vi "MotorBlock_P.vi"(0 "P":dbl, 3 "STOP":bool, 5 "Value":dbl, 7 "Friction Compensation":dbl=0.09 format="%#_13g", 9 "Speed\n (Lower than 900 counts/s)":dbl, 11 "error in (no error)":errorcluster, 12 "Enum":T2(ring), 13 "Motor":T1(ring), 14 "(Antihorario) Sentido (Horario)":bool) -> (4 "Waveform \nChart":dbl[][](graph), 15 "error out":errorcluster)   [LabVIEW 2017]
uses:
  <vilib>/myRIO/Common/Instrument Driver Framework/myRIO v1.0/Encoder/typedefs/Encoder Signal Mode.ctl
  <vilib>/Platform/TimedLoop/XDataNode/timing_clust.ctl
  <vilib>/Platform/TimedLoop/XDataNode/nitl_modes.ctl
  <vilib>/Platform/TimedLoop/XDataNode/wakeup.ctl
  <vilib>/myRIO/Common/Instrument Driver Framework/myRIO v1.0/UART/vis/myRIO v1.0 Close UART.vi
  <vilib>/Utility/error.llb/Error Cluster From Error Code.vi
  <vilib>/myRIO/Common/Instrument Driver Framework/myRIO v1.0/Encoder/vis/myRIO v1.0 Read Encoder.vi
  <vilib>/myRIO/Common/Instrument Driver Framework/myRIO v1.0/DIO/vis/myRIO v1.0 Write DIO.vi
  <vilib>/myRIO/Common/Instrument Driver Framework/myRIO v1.0/PWM/vis/myRIO v1.0 Write PWM.vi
  <vilib>/myRIO/Common/Instrument Driver Framework/Utilities/vis/FPGA Ref Manager.vi
  <vilib>/myRIO/Common/Instrument Driver Framework/myRIO v1.0/myRIO v1.0 Reset FPGA.vi
  <vilib>/myRIO/Common/Instrument Driver Framework/myRIO v1.0/IRQ/vis/myRIO v1.0 IRQ Info FGV.vi
  <vilib>/myRIO/Common/Instrument Driver Framework/myRIO v1.0/IRQ/vis/myRIO v1.0 Timer IRQ Info FGV.vi
  <vilib>/myRIO/Common/Instrument Driver Framework/myRIO v1.0/IRQ/vis/myRIO v1.0 ISR Agent.vi
  <vilib>/Platform/TimedLoop/XDataNode/XDataNode.xnode
  <vilib>/myRIO/Instrument Drivers/Onboard IO/Encoder/Encoder.lvlib
  <vilib>/myRIO/Instrument Drivers/Onboard IO/DIO/DIO.lvlib
  <vilib>/myRIO/Instrument Drivers/Onboard IO/PWM/PWM.lvlib
  <vilib>/myRIO/Instrument Drivers/Utilities/Utilities.lvlib
  <vilib>/Platform/TimedLoop/XDataNode/XDNodeRunTimeDep.lvlib
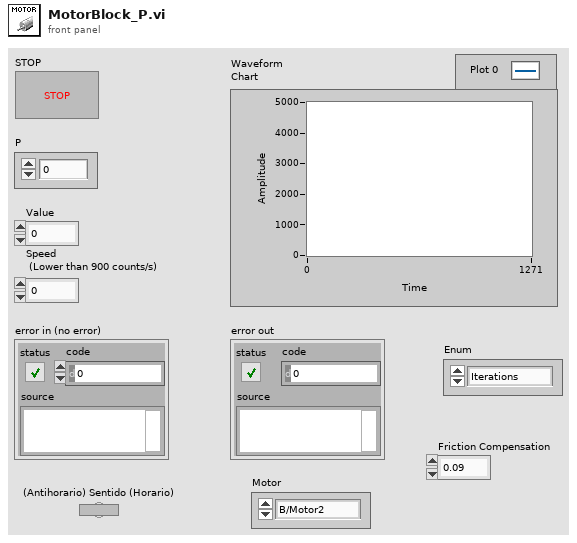
[diagram p1: front panel]
types:
  T1 = enum16{"B/Motor2", "B/Motor1", "A/Motor2", "A/Motor1"}
  T2 = enum16{"Iterations", "Rotations", "Counts", "Degrees", "Time"}
  T3 = typedef "Encoder Signal Mode.ctl" = enum16{"Quadrature phase signal", "Step and direction signal"}
  T4 = typedef "XDNodeRunTimeDep.lvlib/timing_clust.ctl" = cluster{"Expected End [f-1]":u64, "Actual End [f-1]":u64, "Finished Late? [f-1]":bool, "Expected End [i-1]":u64, "Actual End [i-1]":u64, "Finished Late? [i-1]":bool, "Expected Start [i]":u64, "Actual Start [i]":u64, "Expected Start [f]":u64, "Actual Start [f]":u64, "Source Name":string, "Structure Name":string, "Period":i64, "Deadline":i64, "Offset":i64, "Start":i64, "Priority":i32, "Timeout":i32, "Mode":T5, "Wakeup Reason":T6, "Error":errorcluster, "Source Type":string, "Secondary Source Type":string, "Global End Time":u64, "Global Start Time":u64, "Frame Duration":u64, "Iteration Duration":u64, "Assigned CPU":i32, "I/O Scan Engine Mode":u32}
  T5 = typedef "XDNodeRunTimeDep.lvlib/nitl_modes.ctl" = enum32{"No Change", "Process missed periods, maintain original phase", "Discard missed periods, maintain original phase", "Process missed periods, ignore original phase", "Discard missed periods, ignore original phase"}
  T6 = typedef "XDNodeRunTimeDep.lvlib/wakeup.ctl" = enum32{"Normal", "Aborted", "Asynchronous wakeup", "Timing source error", "Timed loop error", "Timeout"}
  T7 = typedef "Encoder.lvlib/Encoder Reference.ctl" = cluster{"myRIO Reference":T8, "Encoder Channels Enum":T12}
  T8 = typedef "myRIO Generic Hardware Reference.ctl" = cluster{"myRIO Model":T9, "myRIO Hardware Reference":T10}
  T9 = typedef "Hardware Version Enum.ctl" = enum16{"Unknown", "myRIO-1900", "myRIO-1950", "roboRIO", "NI ELVIS RIO CM"}
  T10 = typedef "myRIO v1.0 Reference.ctl" = cluster{"Generic FPGA Reference":T11, "Allow multiple opens":bool}
  T11 = typedef "Generic FPGA Reference.ctl" = refnum<k20>
  T12 = typedef "Encoder Channels Enum.ctl" = enum16{"Not Connected", "C/ENC0", "C/ENC1", "A/ENC", "B/ENC", "DIO/ENC0", "DIO/ENC1", "DIO/ENC2", "DIO/ENC3", "DIO/ENC4"}
  T13 = typedef "DIO.lvlib/DIO Reference.ctl" = cluster{"myRIO Reference":T8, "DIO Channels List":T14}
  T14 = typedef "DIO Channels List.ctl" = T15[]
  T15 = typedef "DIO Channels Enum.ctl" = enum16{"Not Connected", "C/DIO0", "C/DIO1", "C/DIO2", "C/DIO3", "C/DIO4", "C/DIO5", "C/DIO6", "C/DIO7", "A/DIO0", "A/DIO1", "A/DIO2", "A/DIO3", "A/DIO4", "A/DIO5", "A/DIO6", "A/DIO7", "A/DIO8", "A/DIO9", "A/DIO10", "A/DIO11", "A/DIO12", "A/DIO13", "A/DIO14", "A/DIO15", "B/DIO0", "B/DIO1", "B/DIO2", "B/DIO3", "B/DIO4", "B/DIO5", "B/DIO6", "B/DIO7", "B/DIO8", "B/DIO9", "B/DIO10", "B/DIO11", "B/DIO12", "B/DIO13", "B/DIO14", "B/DIO15", "LED0", "LED1", "LED2", "LED3", "Button0", "DIO/DIO0", "DIO/DIO1", "DIO/DIO2", "DIO/DIO3", "DIO/DIO4", "DIO/DIO5", "DIO/DIO6", "DIO/DIO7", "DIO/DIO8", "DIO/DIO9", "SPI/CS0", "SPI/CS1", "SPI/CS2", "SPI/CS3", "LED RADIO (Green)", "LED RADIO (Red)", "LED COMM (Green)", "LED COMM (Red)", "LED MODE (Green)", "LED MODE (Red)"}
  T16 = typedef "PWM.lvlib/PWM Reference.ctl" = cluster{"myRIO Reference":T8, "PWM Channels Enum":T17, "PWM Configuration":T18}
  T17 = typedef "PWM Channels Enum.ctl" = enum16{"Not Connected", "C/PWM0", "C/PWM1", "A/PWM0", "A/PWM1", "A/PWM2", "B/PWM0", "B/PWM1", "B/PWM2", "PWM/PWM0", "PWM/PWM1", "PWM/PWM2", "PWM/PWM3", "PWM/PWM4", "PWM/PWM5", "PWM/PWM6", "PWM/PWM7", "PWM/PWM8", "PWM/PWM9"}
  T18 = typedef "PWM.lvlib/PWM Configuration.ctl" = cluster{"Frequency":dbl, "Duty Cycle":dbl}
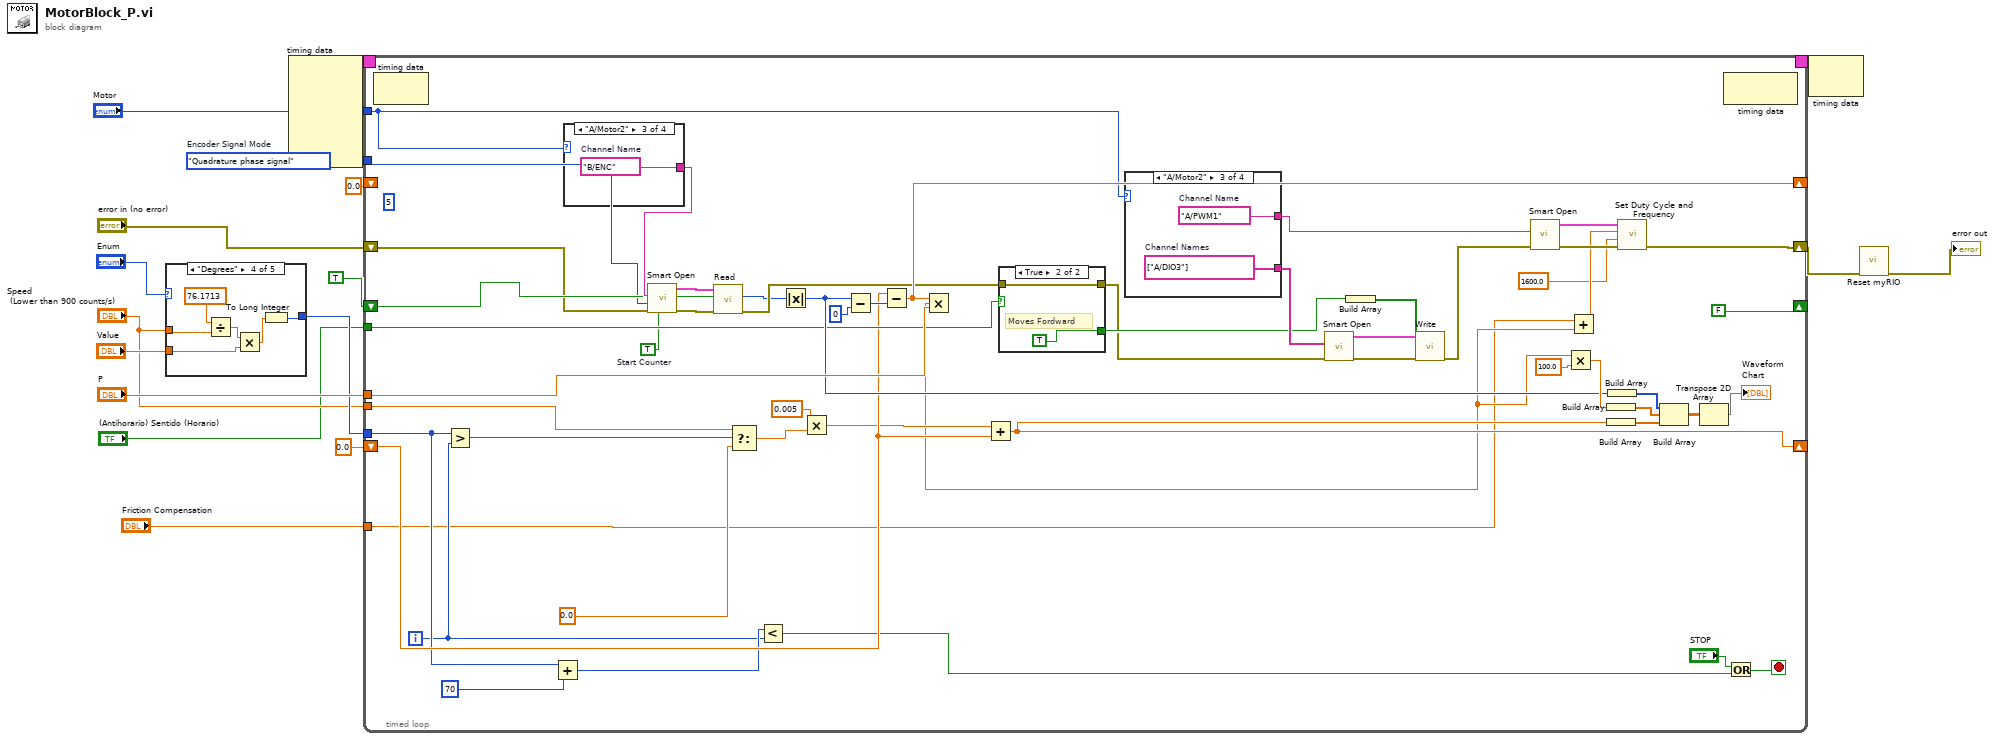
[diagram p0: block diagram]
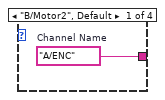
[diagram p2: hidden frame]
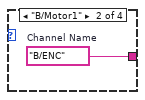
[diagram p3: hidden frame]
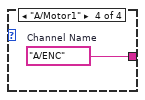
[diagram p4: hidden frame]
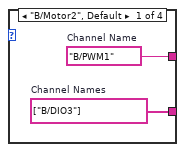
[diagram p5: hidden frame]
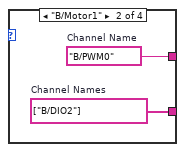
[diagram p6: hidden frame]
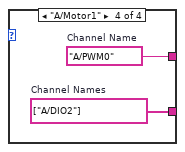
[diagram p7: hidden frame]
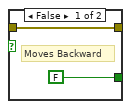
[diagram p8: hidden frame]
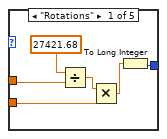
[diagram p9: hidden frame]
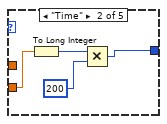
[diagram p10: hidden frame]
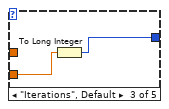
[diagram p11: hidden frame]
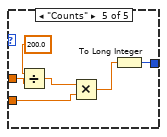
[diagram p12: hidden frame]
diagram:
  w4 = Encoder_Signal_Mode."Quadrature phase signal"  # Encoder Signal Mode
  n1 = case shown="\"Degrees\"" "Enum" {
    tunnel: "Value" -> [w19 w24 w29 w30 w37]
    tunnel: "Speed\n (Lower than 900 counts/s)" -> [w20 _ _ w33 w40]
    tunnel: [w18 w26 w28 w35 w41] -> w10
    frame "Rotations" {
      n2 = Divide(x=27421.68 ("y"), y=w20) -> (x/y=w23:dbl)
      n3 = Multiply(x=w23, y=w19) -> (x*y=w21:dbl)
      n4 = To Long Integer(number=w21) -> (32bit integer=w18:i32)
    }
    frame "Time" {
      n5 = To Long Integer(number=w24) -> (32bit integer=w25:i32)
      n6 = Multiply(x=w25, y=200) -> (x*y=w26:i32)
    }
    frame "Iterations", Default {
      n7 = To Long Integer(number=w29) -> (32bit integer=w28:i32)
    }
    frame "Degrees" {
      n8 = Divide(x=76.1713 ("y"), y=w33) -> (x/y=w31:dbl)
      n9 = Multiply(x=w31, y=w30) -> (x*y=w34:dbl)
      n10 = To Long Integer(number=w34) -> (32bit integer=w35:i32)
    }
    frame "Counts" {
      n11 = Divide(x=200.0, y=w40) -> (x/y=w38:dbl)
      n12 = Multiply(x=w38, y=w37) -> (x*y=w36:dbl)
      n13 = To Long Integer(number=w36) -> (32bit integer=w41:i32)
    }
  }
  n14 = node-c288() -> (w2:T4)  [unwired: 6 in]
  n15 = timed-loop {
    shift-right: [w91] -> _
    shift-left: 0.0 -> [w76]
    shift-right: [FALSE] -> _
    shift-left: TRUE -> [w47]
    tunnel: "P" -> [w92]
    shift-right: [w85] -> _
    shift-left: 0.0 -> [_]
    tunnel: "Speed\n (Lower than 900 counts/s)" -> [w87]
    shift-right: [w60] -> w5
    shift-left: "error in (no error)" -> [w42]
    tunnel: w10 -> [w71]
    tunnel: "(Antihorario) Sentido (Horario)" -> [w77]
    tunnel: "Motor" -> [w49]
    tunnel: w4 -> [w44]
    tunnel: "Friction Compensation" -> [w43]
    timing: w2 -> [_]
    timing-out: [_] -> w1
    i -> [w68]
    stop <- w72 stop-if-true
    w52 = TRUE  # Start Counter
    (unwired) 5
    n16 = node-c288() -> ()  [unwired: 1 in, 1 out]
    n17 = Greater?(x=w71, y=w68) -> (0:w81:bool)
    n18 = Add(x=w71, y=70) -> (x+y=w69:i32)
    n19 = case shown="\"A/Motor2\"" w49 {
      tunnel: [w98 w99 w100 w101] -> w48
      frame "B/Motor2", Default {
        w98 = tag "A/ENC"  # Channel Name
      }
      frame "B/Motor1" {
        w99 = tag "B/ENC"  # Channel Name
      }
      frame "A/Motor2" {
        w100 = tag "B/ENC"  # Channel Name
      }
      frame "A/Motor1" {
        w101 = tag "A/ENC"  # Channel Name
      }
    }
    n20 = call <vilib>:"Smart Open.vi"("Start Counter"=w52, "error in (no error)"=w42, "Encoder Signal Mode"=w44, "Channel Name"=w48) -> ("error out"=w50:errorcluster, "Encoder Ref Out"=w51:T7)  [unwired: 6 in]
    n21 = call <vilib>:"Read.vi"("error in (no error)"=w50, "Reset Counter"=w47, "Encoder Ref In"=w51) -> ("error out"=w46:errorcluster, "Counter Value"=w45:i32)  [unwired: 4 in, 3 out]
    n22 = Select(t=w87, s=w81, f=0.0) -> (s? t:f=w95:dbl)
    n23 = Less?(x=w69, y=w68) -> (x < y?=w73:bool)
    n24 = Absolute Value(x=w45) -> (abs(x)=w78:i32)
    n25 = Multiply(x=0.005 ("y"), y=w95) -> (x*y=w75:dbl)
    n26 = Subtract(x=w78, y=0) -> (x-y=w80:i32)
    n27 = Subtract(x=w76, y=w80) -> (x-y=w85:dbl)
    n28 = Multiply(x=w85, y=w92) -> (x*y=w66:dbl)
    n29 = Add(x=w75, y=w76) -> (x+y=w91:dbl)
    n30 = case shown="True" w77 {
      tunnel: w46 -> [w110 w112]
      tunnel: [FALSE ("A/DIO3 (Pin 17)") TRUE ("A/DIO3 (Pin 17)")] -> w55
      tunnel: [w110 w112] -> w54
      frame False {
        # "Moves Backward"
      }
      frame True {
        # "Moves Fordward"
      }
    }
    n31 = case shown="\"A/Motor2\"" w49 {
      tunnel: [w102 w105 w106 w109] -> w63
      tunnel: [w103 w104 w107 w108] -> w56
      frame "B/Motor2", Default {
        w103 = tag[] ["B/DIO3"]  # Channel Names
        w102 = tag "B/PWM1"  # Channel Name
      }
      frame "B/Motor1" {
        w104 = tag[] ["B/DIO2"]  # Channel Names
        w105 = tag "B/PWM0"  # Channel Name
      }
      frame "A/Motor2" {
        w107 = tag[] ["A/DIO3"]  # Channel Names
        w106 = tag "A/PWM1"  # Channel Name
      }
      frame "A/Motor1" {
        w108 = tag[] ["A/DIO2"]  # Channel Names
        w109 = tag "A/PWM0"  # Channel Name
      }
    }
    n32 = call <vilib>:"Smart Open.vi"("error in (no error)"=w54, "Channel Names"=w56) -> ("error out"=w59:errorcluster, "DIO Ref Out"=w58:T13)  [unwired: 8 in]
    n33 = Build Array(w55) -> (w57:bool[])
    n34 = call <vilib>:"Write.vi"("error in (no error)"=w59, "Values"=w57, "DIO Ref In"=w58) -> ("error out"=w53:errorcluster)  [unwired: 6 in, 1 out]
    n35 = call <vilib>:"Smart Open.vi"("error in (no error)"=w53, "Channel Name"=w63) -> ("error out"=w64:errorcluster, "PWM Ref Out"=w65:T16)  [unwired: 8 in]
    n36 = Multiply(x=w66, y=100.0) -> (x*y=w82:dbl)
    n37 = Add(x=w43, y=w66) -> (x+y=w62:dbl)
    n38 = Build Array(w82) -> (w86:dbl[])
    n39 = Build Array(w91) -> (w90:dbl[])
    n40 = Build Array(w78) -> (w89:i32[])
    n41 = call <vilib>:"Set Duty Cycle and Frequency.vi"("error in (no error)"=w64, "Frequency [Hz]"=1600.0 ("Duty Cycle"), "Duty Cycle"=w62, "PWM Ref In"=w65) -> ("error out"=w60:errorcluster)  [unwired: 5 in, 1 out]
    n42 = Build Array(w89, w86, w90) -> (w88:dbl[][])
    n43 = Transpose 2D Array(2D array=w88) -> (transposed array=→"Waveform \nChart":dbl[][])
    n44 = node-c288() -> ()  [unwired: 1 in, 1 out]
    n45 = Or(x="STOP", y=w73) -> (x .or. y?=w72:bool)
  }
  n46 = node-c288(w1) -> ()  [unwired: 1 out]
  n47 = call <vilib>:"Reset myRIO.vi"("error in (no error)"=w5) -> ("error out"=→"error out":errorcluster)  [unwired: 10 in]
